vi "3D-CollectErrorCodeMessage.vi"(8 "Codemessage":string, 11 "ErrorMessage":string[](array[string])) -> (3 "Error Code Message":string)   [LabVIEW 2017]
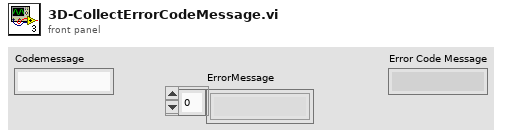
[diagram p1: front panel]
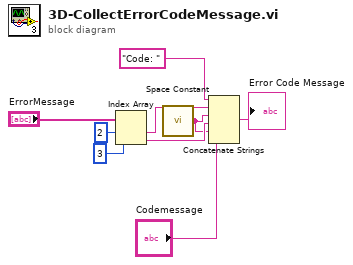
[diagram p0: block diagram]
diagram:
  n1 = Index Array(array="ErrorMessage", index #1=2 ("索引"), index #2=3 ("索引")) -> (element #1=w5:string, element #2=w4:string)
  n2 = call <vilib>:"Space Constant.vi"() -> ("String"=w1:string)
  n3 = Concatenate Strings("Code: ", w5, w1, w4, w1, "Codemessage") -> (→"Error Code Message":string)
